vi "2048_main.vi"() -> ()   [LabVIEW 2022 SP3]
uses:
  gameover.ctl
panel:
  out "end with no movable steps":bool
  out "movable steps":dbl
  out "Challenge steps":dbl[](array[numeric])
  in  "Challenge Mode":bool
  in  "AI  Open":bool
  in  "module path 3":path
  out "error out 3":errorcluster
  out "output cluster 3":cluster{"Score":i32, "Array out":i32[][]}
  out "title 2":string
  in  "gameover 2":T1
  out "Board 2":u16[][](array[ring])
  out "Score":i32
  in  "first bgm 2":path
  in  "target 3 bgm":path
  in  "first bgm":path
  in  "target 1 bgm":path
  in  "target 2 bgm":path
  in  "found target?":bool
  in  "idx":dbl
  out "Array":dbl[](array[numeric])
  in  "AI  mode":bool
  out "output cluster":cluster{"Score":i32, "Array out":i32[][]}
  out "error out":errorcluster
  in  "module path":path
  out "Numeric":i32
  out "title":string
  in  "gameover":T1
  in  "new game":bool
  out "Score":i32
  in  "stop":bool
  out "Board":u16[][](array[ring])
  out "summon_ani 2":u16[][](array[ring]) caption="Ring"
  out "summon_ani":u16[][](array[ring]) caption="Ring"
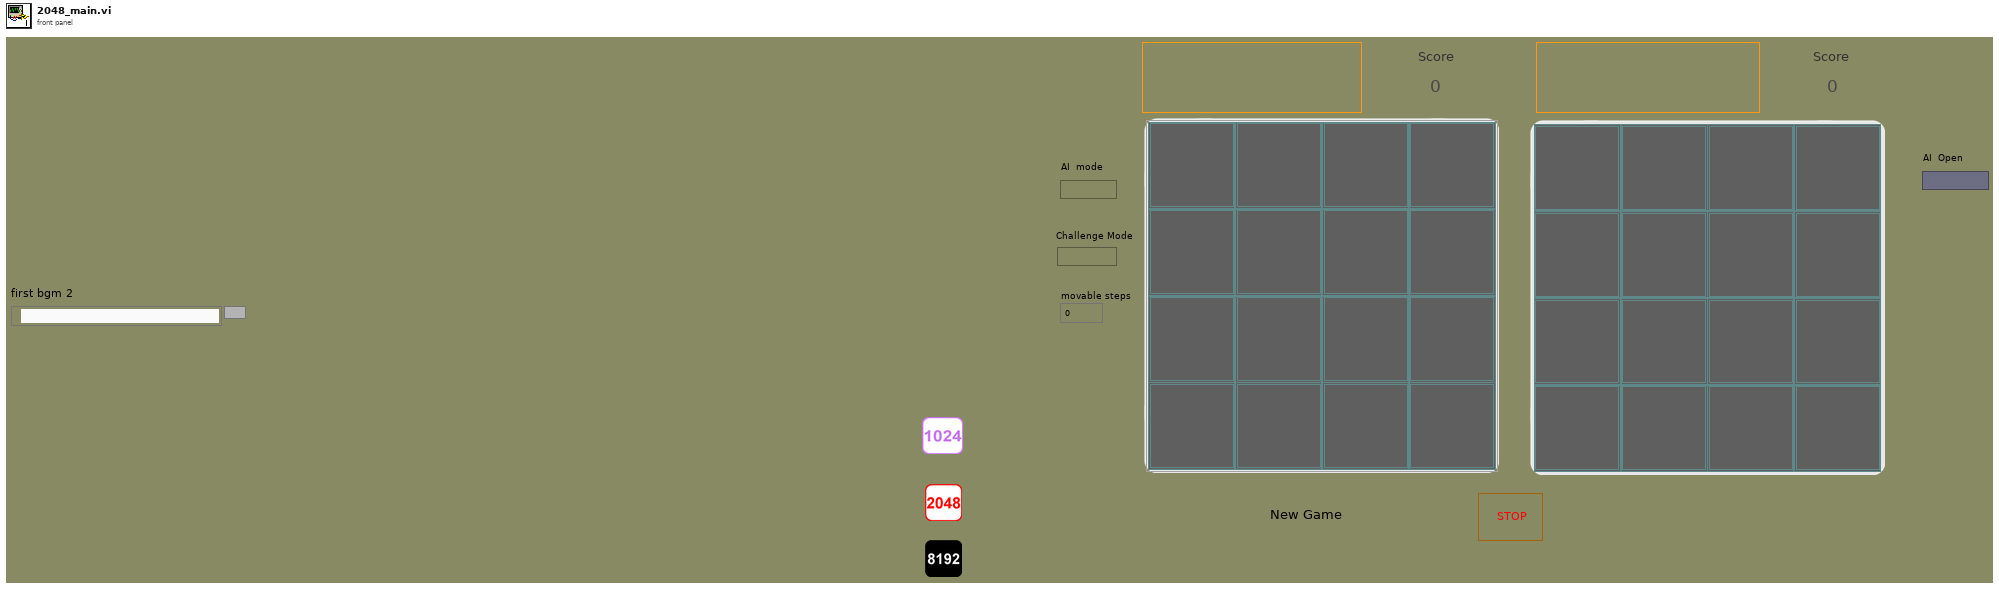
[diagram p1: front panel]
types:
  T1 = typedef "gameover.ctl" = bool
  T2 = typedef "eventvkey.ctl" = enum16{"ASCII", "Enter", "Return", "Shift", "Ctrl", "Alt", "Cmd", "Opt", "Caps", "NumLock", "Clear", "Break", "Up", "Down", "Left", "Right", "Insert", "Delete", "Home", "End", "PageUp", "PageDown", "Escape", "Help", "Pause", "ScrollLock", "F1", "F2", "F3", "F4", "F5", "F6", "F7", "F8", "F9", "F10", "F11", "F12", "F13", "F14", "F15", "F16", "F17", "F18", "F19", "F20", "F21", "F22", "F23", "F24", "Play", "VolumeUp", "VolumeDown", "Mute", "Two Byte Char"}
  T3 = typedef "Sound Output Task ID.ctl" = u32
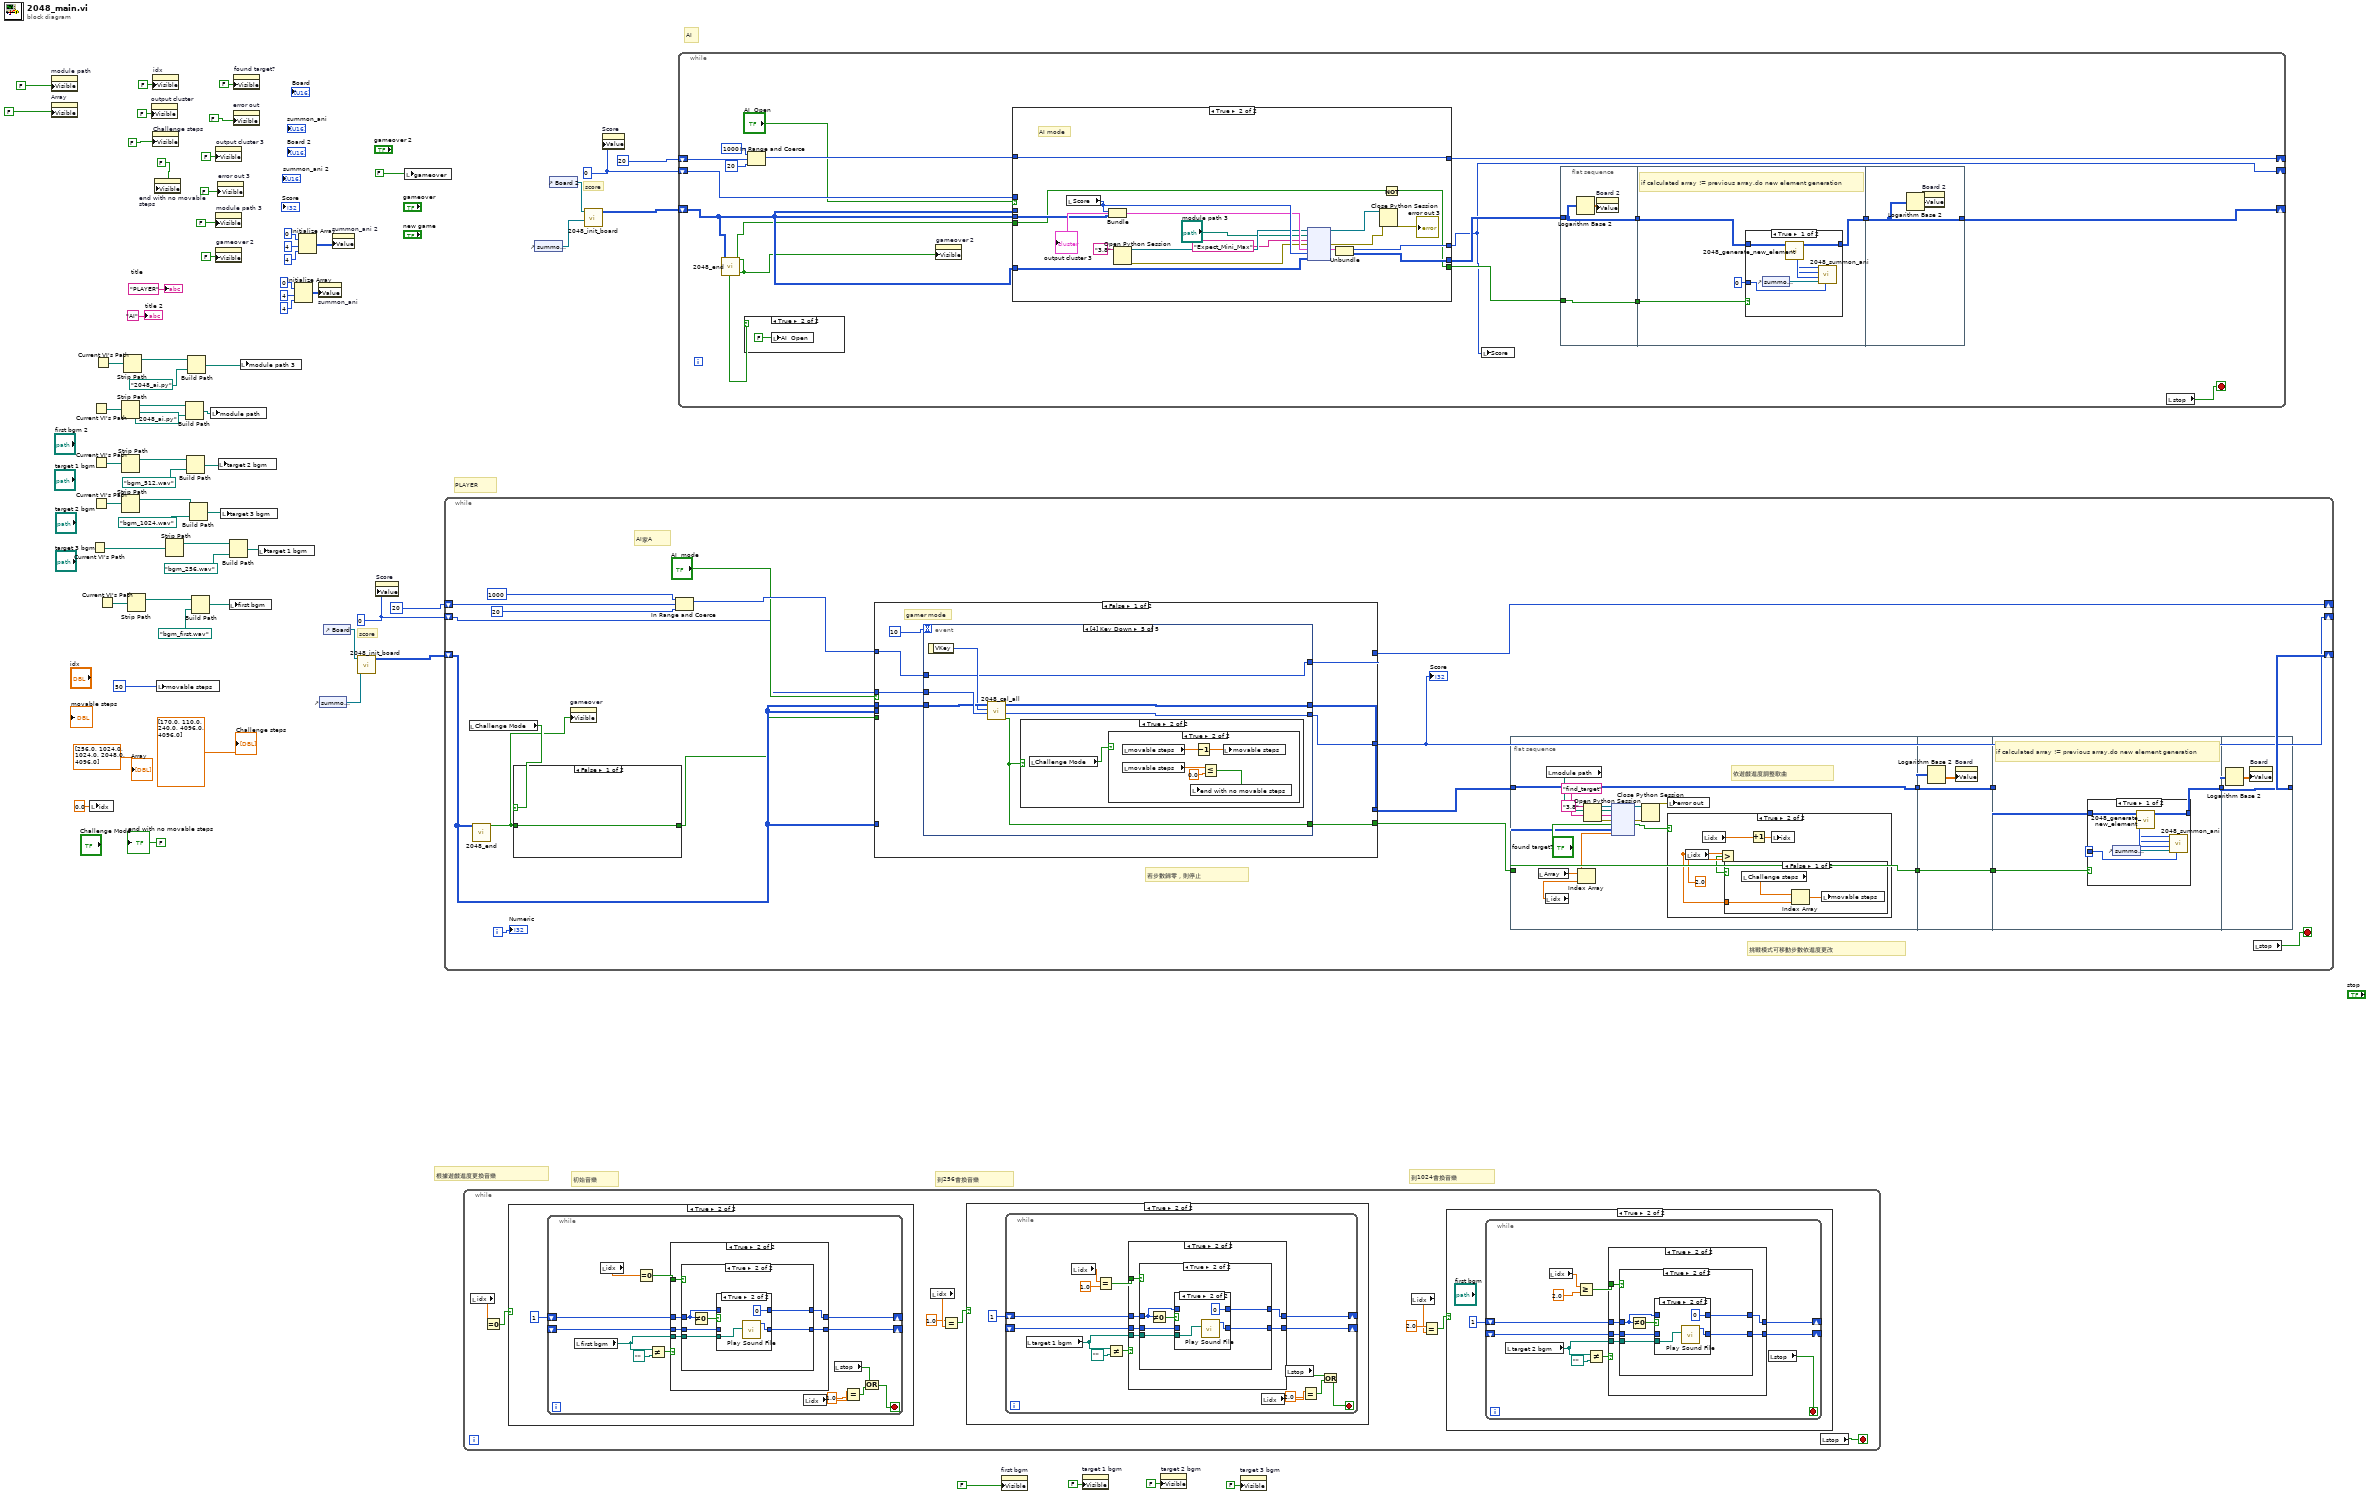
[diagram p0: block diagram]
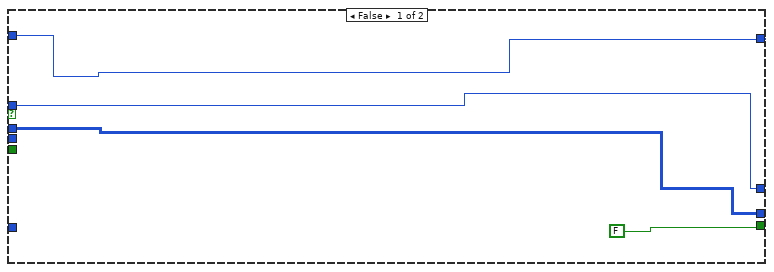
[diagram p3: hidden frame]
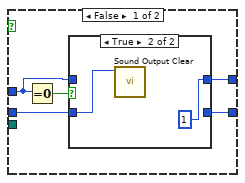
[diagram p7: hidden frame]
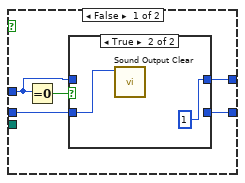
[diagram p12: hidden frame]
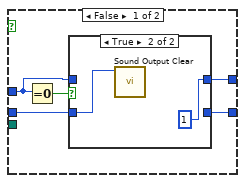
[diagram p17: hidden frame]
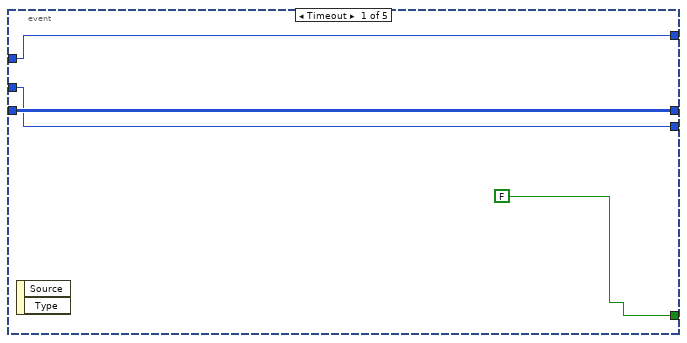
[diagram p20: hidden frame]
diagram:
  w23 = 0
  w58 = 0
  # "PLAYER"
  # "AI"
  # "初始音樂"
  # "到1024會換音樂"
  # "到256會換音樂"
  # "score"
  # "根據遊戲進度更換音樂"
  # "score"
  n1 = property on="module path" class="Path"("Visible"=FALSE) -> ()  [unwired: 2 in, 2 out]
  n2 = property on="Array" class="Arr (strict)"("Visible"=FALSE) -> ()  [unwired: 2 in, 2 out]
  n3 = local write "idx"(0.0 ("idx")) -> ()
  n4 = Current VI's Path() -> (path=w50:path)
  n5 = Current VI's Path() -> (path=w39:path)
  n6 = Current VI's Path() -> (path=w41:path)
  n7 = Current VI's Path() -> (path=w47:path)
  n8 = Current VI's Path() -> (path=w13:path)
  n9 = Current VI's Path() -> (path=w55:path)
  n10 = Strip Path(path=w39) -> (stripped path=w38:path)  [unwired: 1 out]
  n11 = Strip Path(path=w41) -> (stripped path=w42:path)  [unwired: 1 out]
  n12 = Strip Path(path=w47) -> (stripped path=w46:path)  [unwired: 1 out]
  n13 = Strip Path(path=w13) -> (stripped path=w14:path)  [unwired: 1 out]
  n14 = Strip Path(path=w55) -> (stripped path=w54:path)  [unwired: 1 out]
  n15 = property on="output cluster" class="Clust (strict)"("Visible"=FALSE) -> ()  [unwired: 2 in, 2 out]
  n16 = property on="idx" class="DigNum (strict)"("Visible"=FALSE) -> ()  [unwired: 2 in, 2 out]
  n17 = property on="Challenge steps" class="Arr (strict)"("Visible"=FALSE) -> ()  [unwired: 2 in, 2 out]
  n18 = property on="end with no movable steps" class="Bool (strict)"("Visible"=FALSE) -> ()  [unwired: 2 in, 2 out]
  n19 = local write "movable steps"(50) -> ()
  n20 = Strip Path(path=w50) -> (stripped path=w51:path)  [unwired: 1 out]
  n21 = Build Path(base path=w38, name or relative path=path "2048_ai.py") -> (appended path=w36:path)
  n22 = Build Path(base path=w46, name or relative path=path "bgm_512.wav") -> (appended path=w44:path)
  n23 = Build Path(base path=w14, name or relative path=path "2048_ai.py") -> (appended path=w12:path)
  n24 = Build Path(base path=w42, name or relative path=path "bgm_1024.wav") -> (appended path=w40:path)
  n25 = Build Path(base path=w54, name or relative path=path "bgm_first.wav") -> (appended path=w52:path)
  n26 = local write "module path"(w36) -> ()
  n27 = property on="output cluster 3" class="Clust (strict)"("Visible"=FALSE) -> ()  [unwired: 2 in, 2 out]
  n28 = property on="module path 3" class="Path"("Visible"=FALSE) -> ()  [unwired: 2 in, 2 out]
  n29 = property on="gameover 2" class="Bool (strict)"("Visible"=FALSE) -> ()  [unwired: 2 in, 2 out]
  n30 = property on="error out 3" class="Clust (strict)"("Visible"=FALSE) -> ()  [unwired: 2 in, 2 out]
  n31 = local write "target 2 bgm"(w44) -> ()
  n32 = local write "target 3 bgm"(w40) -> ()
  n33 = local write "first bgm"(w52) -> ()
  n34 = Build Path(base path=w51, name or relative path=path "bgm_256.wav") -> (appended path=w48:path)
  n35 = property on="error out" class="Clust (strict)"("Visible"=FALSE) -> ()  [unwired: 2 in, 2 out]
  n36 = property on="found target?" class="Bool (strict)"("Visible"=FALSE) -> ()  [unwired: 2 in, 2 out]
  n37 = local write "module path 3"(w12) -> ()
  n38 = local write "target 1 bgm"(w48) -> ()
  n39 = Initialize Array(0 ("element"), 4 ("dimension size"), 4 ("dimension size")) -> (w66:i32[][])
  n40 = Initialize Array(0 ("element"), 4 ("dimension size"), 4 ("dimension size")) -> (w16:i32[][])
  n41 = property on="summon_ani" class="Arr (strict)"("Value"=w66) -> ()  [unwired: 2 in, 2 out]
  n42 = control-ref of="summon_ani"() -> (w61:refnum<vi>)
  n43 = control-ref of="Board"() -> (w60:refnum<vi>)
  n44 = property on="summon_ani 2" class="Arr (strict)"("Value"=w16) -> ()  [unwired: 2 in, 2 out]
  n45 = call "2048_init_board.vi"("summon_ani"=w61, "Array in"=w60) -> ("Array out"=w59:i32[][])  [unwired: 9 in]
  n46 = property on="Score" class="DigNum (strict)"("Value"=w58) -> ()  [unwired: 2 in, 2 out]
  n47 = local write "gameover"(T1 FALSE ("gameover")) -> ()
  n48 = while {
    shift-right: [w84] -> _
    shift-left: w59 -> [w76]
    shift-right: [w70] -> _
    shift-left: w58 -> [w72]
    shift-right: [w71] -> _
    shift-left: 20 -> [w80]
    i -> [w85]
    stop <- w77 stop-if-true
    # "AI家Α"
    # "若步數歸零，則停止"
    # "挑戰模式可移動步數依進度更改"
    n49 = local read "Challenge Mode"() -> (w74:bool)
    n50 = call "2048_end.vi"("Array in"=w76) -> ("Boolean"=w67:bool)  [unwired: 10 in]
    n51 = case shown="False" w74 {
      tunnel: w67 -> [w148 w150]
      tunnel: [w148 w149] -> w75
      frame False {
      }
      frame True {
        n52 = local read "end with no movable steps"() -> (w151:bool)
        n53 = Or(x=w151, y=w150) -> (x .or. y?=w149:bool)
      }
    }
    n54 = property on="gameover" class="Bool (strict)"("Visible"=w67) -> ()  [unwired: 2 in, 2 out]
    n55 = In Range and Coerce(upper limit=1000, x=w80, lower limit=20) -> (coerced(x)=w81:i32)  [unwired: 1 out]
    n56 = case shown="False" "AI  mode" {
      tunnel: w72 -> [w96 _]
      tunnel: [w95 w130] -> w71
      tunnel: w81 -> [w94 w130]
      tunnel: w76 -> [w93 _]
      tunnel: w76 -> [_ w138]
      tunnel: w75 -> [_ w137]
      tunnel: w76 -> [_ w135]
      tunnel: [w89 w133] -> w70
      tunnel: [w90 w132] -> w69
      tunnel: [w91 w131] -> w68
      frame False {
        # "gamer mode"
        n57 = event shown="[4] Key Down" {
          selector: _ -> [_ _ _ _ _]
          dyn-events: _ -> [_ _ _ _ _]
          timeout: 10 -> [_ _ _ _ _]
          tunnel: [w100 w104 w110 w115 w119] -> w90
          tunnel: w96 -> [w99 _ w109 w114 w123]
          tunnel: w93 -> [w100 _ w110 w115 w122]
          tunnel: [FALSE FALSE ("valid move") FALSE ("valid move") FALSE ("valid move") w117] -> w91
          tunnel: [w99 0 ("score") w109 w114 w121] -> w89
          tunnel: w94 -> [w98 _ w107 w112 w118]
          tunnel: [w98 20 w107 w112 w118] -> w95
          event Timeout {
            n58 = event-data() -> ()  [unwired: 1 in, 2 out]
          }
          event "new game": Mouse Down {
            n59 = event-data() -> ()  [unwired: 1 in, 1 out]
            n60 = control-ref of="summon_ani"() -> (w106:refnum<vi>)
            n61 = control-ref of="Board"() -> (w105:refnum<vi>)
            n62 = call "2048_init_board.vi"("summon_ani"=w106, "Array in"=w105) -> ("Array out"=w104:i32[][])  [unwired: 9 in]
          }
          event "new game": Mouse Enter {
            n63 = event-data() -> ()  [unwired: 1 in, 1 out]
            n64 = property on="new game" class="Bool (strict)"("BoolText.TextColor"=u32 33023 ("Boolean Text.Text Colors:Text Color")) -> ()  [unwired: 2 in, 2 out]
          }
          event "new game": Mouse Leave {
            n65 = event-data() -> ()  [unwired: 1 in, 1 out]
            n66 = property on="new game" class="Bool (strict)"("BoolText.TextColor"=u32 0 ("Boolean Text.Text Colors:Text Color")) -> ()  [unwired: 2 in, 2 out]
          }
          event Key Down {
            n67 = event-data() -> ("VKey"=w120:T2)  [unwired: 1 in]
            n68 = call "2048_cal_all.vi"("score in"=w123, "VKey in"=w120, "matrix"=w122) -> ("valid move"=w117:bool, "score out"=w121:i32, "matrix out"=w119:i32[][])  [unwired: 5 in, 1 out]
            n69 = case shown="True" w117 {
              frame False {
              }
              frame True {
                n70 = local read "Challenge Mode"() -> (w124:bool)
                n71 = case shown="True" w124 {
                  frame False {
                  }
                  frame True {
                    n72 = local read "movable steps"() -> (w129:dbl)
                    n73 = local read "movable steps"() -> (w127:dbl)
                    n74 = Decrement(x=w129) -> (x-1=w128:dbl)
                    n75 = Less Or Equal?(x=w127, y=0.0) -> (x <= y?=w125:bool)
                    n76 = local write "end with no movable steps"(w125) -> ()
                    n77 = local write "movable steps"(w128) -> ()
                  }
                }
              }
            }
          }
        }
      }
      frame True {
        # "AI mode"
        n78 = local read "Score"() -> (w147:i32)
        n79 = Bundle("Score"=w147, "Array out"=w138) -> (w146:cluster{"Score":i32, "Array out":i32[][]})  [unwired: 1 in]
        "output cluster" <- w146
        n80 = Open Python Session(python version="3.8" ("Python version")) -> (session out=w140:refnum<k35>, error out=w141:errorcluster)  [unwired: 2 in]
        n81 = node(w140, "module path", "Expect_Mini_Max" ("function name"), w141, w146, w147, w135) -> (w145:refnum<k35>, w143:errorcluster, w142:cluster{"Score":i32, "Array out":i32[][]})  [unwired: 2 in, 2 out]
        n82 = Unbundle(w142) -> ("Score"=w133:i32, "Array out"=w132:i32[][])
        n83 = Close Python Session(session in=w145, error in=w143) -> (11:→"error out":errorcluster)
        n84 = Not(x=w137) -> (.not. x?=w131:bool)
      }
    }
    "Score" <- w70
    n85 = flat-sequence {
      tunnel: w68 -> [w166]
      tunnel: w69 -> [w153]
      tunnel: [w153] -> w79
      tunnel: [w166] -> w78
      tunnel: [w177] -> w88
      tunnel: [w176] -> w87
      tunnel: w79 -> [w176]
      tunnel: w78 -> [w177]
      tunnel: w88 -> [w182]
      tunnel: w87 -> [w181]
      tunnel: [w180] -> w86
      tunnel: w86 -> [w191]
      tunnel: [w191] -> w84
      frame #0 {
        # "依遊戲進度調整歌曲"
        n86 = local read "Array"() -> (w163:dbl[])
        n87 = local read "idx"() -> (w164:dbl)
        n88 = local read "module path"() -> (w157:path)
        n89 = Index Array(array=w163, index=w164) -> (element=w165:dbl)
        n90 = Open Python Session(python version="3.8" ("Python version")) -> (session out=w156:refnum<k35>, error out=w155:errorcluster)  [unwired: 2 in]
        n91 = node(w156, w157, "find_target" ("function name"), w155, "found target?", w153, w165) -> (w160:refnum<k35>, w161:errorcluster, w159:bool)  [unwired: 2 in, 2 out]
        n92 = Close Python Session(session in=w160, error in=w161) -> (11:w162:errorcluster)
        n93 = local write "error out"(w162) -> ()
        n94 = case shown="True" w159 {
          frame False {
          }
          frame True {
            n95 = local read "idx"() -> (w167:dbl)
            n96 = local read "idx"() -> (w170:dbl)
            n97 = Greater?(x=w167, y=2.0) -> (0:w168:bool)
            n98 = case shown="False" w168 {
              tunnel: w167 -> [w172 _]
              frame False {
                n99 = local read "Challenge steps"() -> (w173:dbl[])
                n100 = Index Array(array=w173, index=w172) -> (element=w174:dbl)
                n101 = local write "movable steps"(w174) -> ()
              }
              frame True {
                n102 = local write "movable steps"(4096) -> ()
              }
            }
            n103 = Increment(x=w170) -> (x+1=w171:dbl)
            n104 = local write "idx"(w171) -> ()
          }
        }
      }
      frame #1 {
        n105 = Logarithm Base 2(1:w176) -> (0:w178:dbl[][])
        n106 = property on="Board" class="Arr (strict)"("Value"=w178) -> ()  [unwired: 2 in, 2 out]
      }
      frame #2 {
        # "if calculated array != previous array,do new element generation"
        n107 = case shown="True" w182 {
          tunnel: w181 -> [w189 w190]
          tunnel: [w188 w190] -> w180
          tunnel: 0 -> [w187 _]
          frame True {
            n108 = control-ref of="summon_ani"() -> (w186:refnum<vi>)
            n109 = call "2048_generate_new_element.vi"("Array in"=w189) -> ("c"=w185:u64, "r"=w184:u64, "element"=w183:i16, "Array out"=w188:i32[][])  [unwired: 7 in]
            n110 = call "2048_summon_ani.vi"("speed"=w187, "Array in"=w186, "c"=w185, "r"=w184, "element"=w183) -> ()  [unwired: 7 in]
          }
          frame False {
          }
        }
      }
      frame #3 {
        n111 = Logarithm Base 2(1:w191) -> (0:w192:dbl[][])
        n112 = property on="Board" class="Arr (strict)"("Value"=w192) -> ()  [unwired: 2 in, 2 out]
      }
    }
    n113 = local read "stop"() -> (w77:bool)
    "Numeric" <- w85
  }
  n114 = while {
    stop <- w196 stop-if-true
    n115 = local read "idx"() -> (w200:dbl)
    n116 = Equal To 0?(x=w200) -> (x = 0?=w201:bool)
    n117 = case shown="True" w201 {
      frame False {
      }
      frame True {
        n118 = while {
          shift-right: [w297] -> _
          shift-left: _ -> [w298]
          shift-right: [w295] -> _
          shift-left: 1 -> [w296]
          stop <- w287 stop-if-true
          n119 = local read "first bgm"() -> (w294:path)
          n120 = local read "idx"() -> (w291:dbl)
          n121 = Equal To 0?(x=w291) -> (x = 0?=w290:bool)
          n122 = Not Equal?(x=w294, y=path "") -> (x != y?=w299:bool)
          n123 = case shown="True" w299 {
            tunnel: w290 -> [_ w308]
            tunnel: w298 -> [w302 w306]
            tunnel: [w302 w303] -> w297
            tunnel: w296 -> [w301 w307]
            tunnel: [w301 w305] -> w295
            tunnel: w294 -> [_ w304]
            frame False {
            }
            frame True {
              n124 = case shown="True" w308 {
                tunnel: w307 -> [w310 w319]
                tunnel: w306 -> [w312 w318]
                tunnel: [w311 w320] -> w305
                tunnel: w304 -> [_ w322]
                tunnel: [w309 w321] -> w303
                frame False {
                  n125 = Equal To 0?(x=w310) -> (x = 0?=w313:bool)
                  n126 = case shown="True" w313 {
                    tunnel: w312 -> [w314 w317]
                    tunnel: [w315 1] -> w311
                    tunnel: w310 -> [w315 _]
                    tunnel: [w314 _] -> w309
                    frame False {
                    }
                    frame True {
                      n127 = call <vilib>:"Sound Output Clear.vi"("task ID"=w317) -> ()  [unwired: 10 in, 1 out]
                    }
                  }
                }
                frame True {
                  n128 = Not Equal To 0?(x=w319) -> (x != 0?=w323:bool)
                  n129 = case shown="True" w323 {
                    tunnel: w322 -> [_ w328]
                    tunnel: [w324 w327] -> w321
                    tunnel: [w325 0] -> w320
                    tunnel: w319 -> [w325 _]
                    tunnel: w318 -> [w324 _]
                    frame False {
                    }
                    frame True {
                      n130 = call <vilib>:"Play Sound File.vi"("path"=w328) -> ("task ID"=w327:T3)  [unwired: 9 in, 1 out]
                    }
                  }
                }
              }
            }
          }
          n131 = local read "idx"() -> (w293:dbl)
          n132 = local read "stop"() -> (w288:bool)
          n133 = Equal?(x=w293, y=1.0) -> (x = y?=w289:bool)
          n134 = Or(x=w288, y=w289) -> (x .or. y?=w287:bool)
        }
      }
    }
    n135 = local read "idx"() -> (w199:dbl)
    n136 = Equal?(x=1.0, y=w199) -> (x = y?=w198:bool)
    n137 = case shown="True" w198 {
      frame False {
      }
      frame True {
        n138 = while {
          shift-right: [w254] -> _
          shift-left: _ -> [w255]
          shift-right: [w252] -> _
          shift-left: 1 -> [w253]
          stop <- w243 stop-if-true
          n139 = local read "target 1 bgm"() -> (w251:path)
          n140 = local read "idx"() -> (w248:dbl)
          n141 = Equal?(x=w248, y=1.0) -> (x = y?=w247:bool)
          n142 = Not Equal?(x=w251, y=path "") -> (x != y?=w256:bool)
          n143 = case shown="True" w256 {
            tunnel: w247 -> [_ w265]
            tunnel: w255 -> [w259 w263]
            tunnel: [w259 w260] -> w254
            tunnel: w253 -> [w258 w264]
            tunnel: [w258 w262] -> w252
            tunnel: w251 -> [_ w261]
            frame False {
            }
            frame True {
              n144 = case shown="True" w265 {
                tunnel: w264 -> [w267 w276]
                tunnel: w263 -> [w269 w275]
                tunnel: [w268 w277] -> w262
                tunnel: w261 -> [_ w279]
                tunnel: [w266 w278] -> w260
                frame False {
                  n145 = Equal To 0?(x=w267) -> (x = 0?=w270:bool)
                  n146 = case shown="True" w270 {
                    tunnel: w269 -> [w271 w274]
                    tunnel: [w272 1] -> w268
                    tunnel: w267 -> [w272 _]
                    tunnel: [w271 _] -> w266
                    frame False {
                    }
                    frame True {
                      n147 = call <vilib>:"Sound Output Clear.vi"("task ID"=w274) -> ()  [unwired: 10 in, 1 out]
                    }
                  }
                }
                frame True {
                  n148 = Not Equal To 0?(x=w276) -> (x != 0?=w280:bool)
                  n149 = case shown="True" w280 {
                    tunnel: w279 -> [_ w285]
                    tunnel: [w281 w284] -> w278
                    tunnel: [w282 0] -> w277
                    tunnel: w276 -> [w282 _]
                    tunnel: w275 -> [w281 _]
                    frame False {
                    }
                    frame True {
                      n150 = call <vilib>:"Play Sound File.vi"("path"=w285) -> ("task ID"=w284:T3)  [unwired: 9 in, 1 out]
                    }
                  }
                }
              }
            }
          }
          n151 = local read "idx"() -> (w250:dbl)
          n152 = local read "stop"() -> (w244:bool)
          n153 = Equal?(x=w250, y=2.0) -> (x = y?=w245:bool)
          n154 = Or(x=w244, y=w245) -> (x .or. y?=w243:bool)
        }
      }
    }
    n155 = local read "idx"() -> (w193:dbl)
    n156 = Equal?(x=2.0, y=w193) -> (x = y?=w194:bool)
    n157 = case shown="True" w194 {
      frame False {
      }
      frame True {
        n158 = while {
          shift-right: [w210] -> _
          shift-left: _ -> [w211]
          shift-right: [w208] -> _
          shift-left: 1 -> [w209]
          stop <- w203 stop-if-true
          n159 = local read "target 2 bgm"() -> (w207:path)
          n160 = local read "idx"() -> (w206:dbl)
          n161 = Greater Or Equal?(x=w206, y=2.0) -> (x >= y?=w205:bool)
          n162 = Not Equal?(x=w207, y=path "") -> (x != y?=w212:bool)
          n163 = case shown="True" w212 {
            tunnel: w205 -> [_ w221]
            tunnel: w211 -> [w215 w219]
            tunnel: [w215 w216] -> w210
            tunnel: w209 -> [w214 w220]
            tunnel: [w214 w218] -> w208
            tunnel: w207 -> [_ w217]
            frame False {
            }
            frame True {
              n164 = case shown="True" w221 {
                tunnel: w220 -> [w223 w232]
                tunnel: w219 -> [w225 w231]
                tunnel: [w224 w233] -> w218
                tunnel: w217 -> [_ w235]
                tunnel: [w222 w234] -> w216
                frame False {
                  n165 = Equal To 0?(x=w223) -> (x = 0?=w226:bool)
                  n166 = case shown="True" w226 {
                    tunnel: w225 -> [w227 w230]
                    tunnel: [w228 1] -> w224
                    tunnel: w223 -> [w228 _]
                    tunnel: [w227 _] -> w222
                    frame False {
                    }
                    frame True {
                      n167 = call <vilib>:"Sound Output Clear.vi"("task ID"=w230) -> ()  [unwired: 10 in, 1 out]
                    }
                  }
                }
                frame True {
                  n168 = Not Equal To 0?(x=w232) -> (x != 0?=w236:bool)
                  n169 = case shown="True" w236 {
                    tunnel: w235 -> [_ w241]
                    tunnel: [w237 w240] -> w234
                    tunnel: [w238 0] -> w233
                    tunnel: w232 -> [w238 _]
                    tunnel: w231 -> [w237 _]
                    frame False {
                    }
                    frame True {
                      n170 = call <vilib>:"Play Sound File.vi"("path"=w241) -> ("task ID"=w240:T3)  [unwired: 9 in, 1 out]
                    }
                  }
                }
              }
            }
          }
          n171 = local read "stop"() -> (w203:bool)
        }
      }
    }
    n172 = local read "stop"() -> (w196:bool)
  }
  n173 = control-ref of="summon_ani 2"() -> (w20:refnum<vi>)
  n174 = control-ref of="Board 2"() -> (w21:refnum<vi>)
  n175 = call "2048_init_board.vi"("summon_ani"=w20, "Array in"=w21) -> ("Array out"=w22:i32[][])  [unwired: 9 in]
  n176 = property on="Score" class="DigNum (strict)"("Value"=w23) -> ()  [unwired: 2 in, 2 out]
  n177 = while {
    shift-right: [w342] -> _
    shift-left: w22 -> [w334]
    shift-right: [w330] -> _
    shift-left: w23 -> [w341]
    shift-right: [w340] -> _
    shift-left: 20 -> [w336]
    stop <- w333 stop-if-true
    n178 = call "2048_end.vi"("Array in"=w334) -> ("Boolean"=w329:bool)  [unwired: 10 in]
    n179 = case shown="True" w329 {
      frame False {
      }
      frame True {
        n180 = local write "AI  Open"(FALSE ("AI  mode 2")) -> ()
      }
    }
    n181 = In Range and Coerce(upper limit=1000, x=w336, lower limit=20) -> (coerced(x)=w337:i32)  [unwired: 1 out]
    n182 = property on="gameover 2" class="Bool (strict)"("Visible"=w329) -> ()  [unwired: 2 in, 2 out]
    n183 = case shown="True" "AI  Open" {
      tunnel: w341 -> [w348 _]
      tunnel: [w350 w351] -> w340
      tunnel: w337 -> [w350 w351]
      tunnel: w334 -> [w347 _]
      tunnel: w334 -> [_ w359]
      tunnel: w329 -> [_ w358]
      tunnel: w334 -> [_ w356]
      tunnel: [w348 w354] -> w330
      tunnel: [w347 w353] -> w332
      tunnel: [FALSE w352] -> w331
      frame False {
      }
      frame True {
        # "AI mode"
        n184 = local read "Score"() -> (w368:i32)
        n185 = Bundle("Score"=w368, "Array out"=w359) -> (w367:cluster{"Score ":i32, "Array out":i32[][]})  [unwired: 1 in]
        "output cluster 3" <- w367
        n186 = Open Python Session(python version="3.8" ("Python version")) -> (session out=w361:refnum<k35>, error out=w362:errorcluster)  [unwired: 2 in]
        n187 = node(w361, "module path 3", "Expect_Mini_Max" ("function name"), w362, w367, w368, w356) -> (w366:refnum<k35>, w364:errorcluster, w363:cluster{"Score ":i32, "Array out":i32[][]})  [unwired: 2 in, 2 out]
        n188 = Unbundle(w363) -> ("Score"=w354:i32, "Array out"=w353:i32[][])
        n189 = Close Python Session(session in=w366, error in=w364) -> (11:→"error out 3":errorcluster)
        n190 = Not(x=w358) -> (.not. x?=w352:bool)
      }
    }
    n191 = local write "Score"(w330) -> ()
    n192 = flat-sequence {
      tunnel: [w369] -> w345
      tunnel: [w370] -> w344
      tunnel: w332 -> [w370]
      tunnel: w331 -> [w369]
      tunnel: w345 -> [w375]
      tunnel: w344 -> [w374]
      tunnel: [w373] -> w343
      tunnel: w343 -> [w384]
      tunnel: [w384] -> w342
      frame #0 {
        n193 = Logarithm Base 2(1:w370) -> (0:w371:dbl[][])
        n194 = property on="Board 2" class="Arr (strict)"("Value"=w371) -> ()  [unwired: 2 in, 2 out]
      }
      frame #1 {
        # "if calculated array != previous array,do new element generation"
        n195 = case shown="True" w375 {
          tunnel: w374 -> [w382 w383]
          tunnel: [w381 w383] -> w373
          tunnel: 0 -> [w380 _]
          frame True {
            n196 = control-ref of="summon_ani 2"() -> (w379:refnum<vi>)
            n197 = call "2048_generate_new_element.vi"("Array in"=w382) -> ("c"=w378:u64, "r"=w377:u64, "element"=w376:i16, "Array out"=w381:i32[][])  [unwired: 7 in]
            n198 = call "2048_summon_ani.vi"("speed"=w380, "Array in"=w379, "c"=w378, "r"=w377, "element"=w376) -> ()  [unwired: 7 in]
          }
          frame False {
          }
        }
      }
      frame #2 {
        n199 = Logarithm Base 2(1:w384) -> (0:w385:dbl[][])
        n200 = property on="Board 2" class="Arr (strict)"("Value"=w385) -> ()  [unwired: 2 in, 2 out]
      }
    }
    n201 = local read "stop"() -> (w333:bool)
  }
  n202 = property on="first bgm" class="Path"("Visible"=FALSE) -> ()  [unwired: 2 in, 2 out]
  n203 = property on="target 1 bgm" class="Path"("Visible"=FALSE) -> ()  [unwired: 2 in, 2 out]
  n204 = property on="target 2 bgm" class="Path"("Visible"=FALSE) -> ()  [unwired: 2 in, 2 out]
  n205 = property on="target 3 bgm" class="Path"("Visible"=FALSE) -> ()  [unwired: 2 in, 2 out]
  "title" <- "PLAYER" ("title")
  "Array" <- dbl[] [256.0, 1024.0, 1024.0, 2048.0, 4096.0] ("Array")
  "title 2" <- "AI" ("title")
  "Challenge steps" <- dbl[] [170.0, 110.0, 240.0, 4096.0, 4096.0] ("Array")
  "end with no movable steps" <- FALSE ("end with no movable steps")
